vi "OE1022D Example All Data.vi"() -> ()   [LabVIEW 2022 SP3]
uses:
  <vilib>/Utility/file.llb/Write Delimited Spreadsheet (DBL).vi
panel:
  in  "OE1022D 2":refnum<visa-resource-name> caption="OE1022D"
  in  "Scanner Voltage":i32
  in  "File Path":path
  in  "Data Points":i32
  out "Waveform Chart":dbl[](graph)
  out "θh1 (°) 2":sgl caption="θh1 (deg)" format="%.2f"
  out "Rh1 2":sgl caption="Rh1 (Vrms)" format="%.3p"
  out "Yh1 2":sgl caption="Yh1 (Vrms)" format="%.3p"
  out "Xh1 2":sgl caption="Xh1 (Vrms)" format="%.3p"
  out "Xh2 2":sgl caption="Xh2 (Vrms)" format="%.3p"
  out "Yh2 2":sgl caption="Yh2 (Vrms)" format="%.3p"
  out "Rh2 2":sgl caption="Rh2 (Vrms)" format="%.3p"
  out "噪声 2":sgl caption="Noise(Vrms)" format="%.3p"
  out "频率 (Hz) 2":sgl caption="Freq (Hz)" format="%#.3f"
  out "θ (°) 2":sgl caption="θ (deg)" format="%.2f"
  out "R 2":sgl caption="R (Vrms)" format="%.3p"
  out "Y 2":sgl caption="Y (Vrms)" format="%.3p"
  out "θh2 (°) 2":sgl caption="θh2 (deg)" format="%.2f"
  out "X 2":sgl caption="X (Vrms)" format="%.3p"
  out "Yh1":sgl caption="Yh1 (Vrms)" format="%.3p"
  out "Xh1":sgl caption="Xh1 (Vrms)" format="%.3p"
  out "θh2 (°)":sgl caption="θh2 (deg)" format="%.2f"
  out "Yh2":sgl caption="Yh2 (Vrms)" format="%.3p"
  out "Xh2":sgl caption="Xh2 (Vrms)" format="%.3p"
  out "Rh2":sgl caption="Rh2 (Vrms)" format="%.3p"
  out "θh1 (°)":sgl caption="θh1 (deg)" format="%.2f"
  out "Rh1":sgl caption="Rh1 (Vrms)" format="%.3p"
  out "噪声":sgl caption="Noise(Vrms)" format="%.3p"
  out "频率 (Hz)":sgl caption="Freq (Hz)" format="%#.3f"
  out "θ (°)":sgl caption="θ (deg)" format="%.2f"
  out "Y":sgl caption="Y (Vrms)" format="%.3p"
  out "X":sgl caption="X (Vrms)" format="%.3p"
  out "R":sgl caption="R (Vrms)" format="%.3p"
  out "AUX-ADC2 (V)":sgl format="%.3f"
  out "AUX-ADC1 (V)":sgl format="%.3f"
  out "AUX-ADC3 (V)":sgl format="%.3f"
  out "AUX-ADC4 (V)":sgl format="%.3f"
  out "错误输出":errorcluster
  out "序列号":string
  # "input 0 for continous"
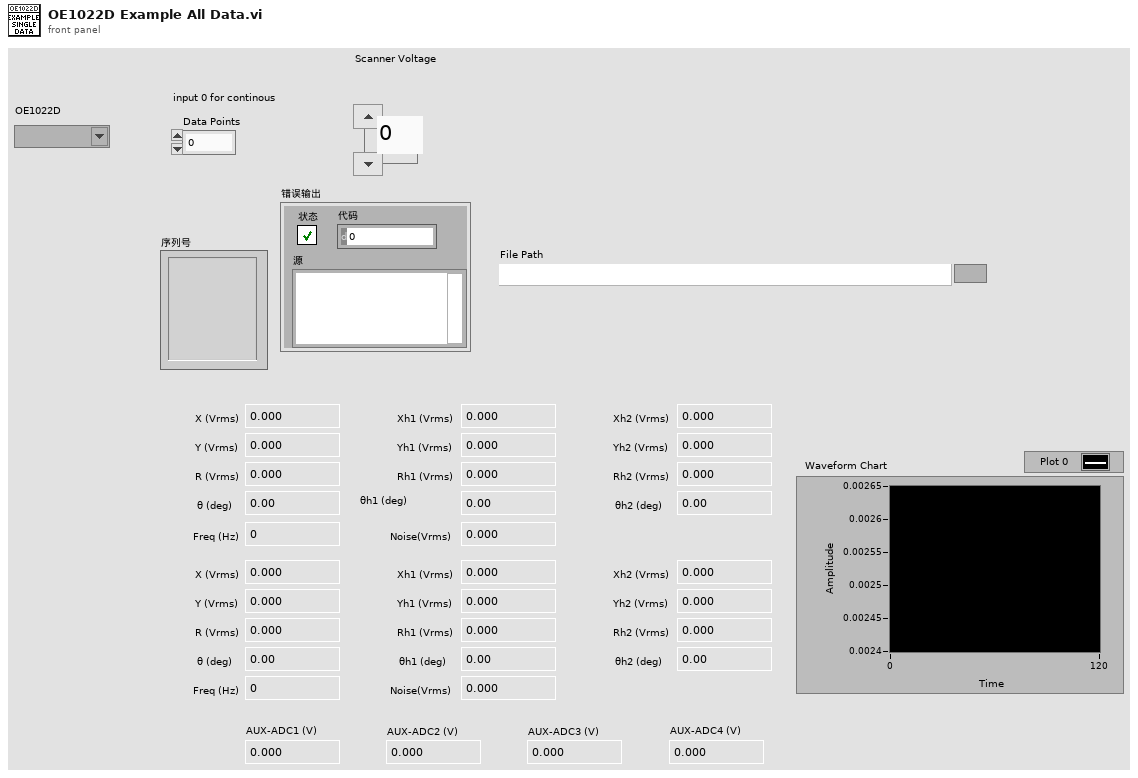
[diagram p1: front panel]
types:
  T1 = cluster{"AD1":dbl[], "AD2":dbl[], "AD3":dbl[], "AD4":dbl[]}
  T2 = cluster{"XB":dbl[], "YB":dbl[], "FrequencyB":dbl[], "NoiseB":dbl[], "Xh1B":dbl[], "Yh1B":dbl[], "Xh2B":dbl[], "Yh2B":dbl[], "Xh2B":dbl[]}
  T3 = cluster{"XA":dbl[], "YA":dbl[], "FrequencyA":dbl[], "NoiseA":dbl[], "Xh1A":dbl[], "Yh1A":dbl[], "Xh2A":dbl[], "Yh2A":dbl[]}
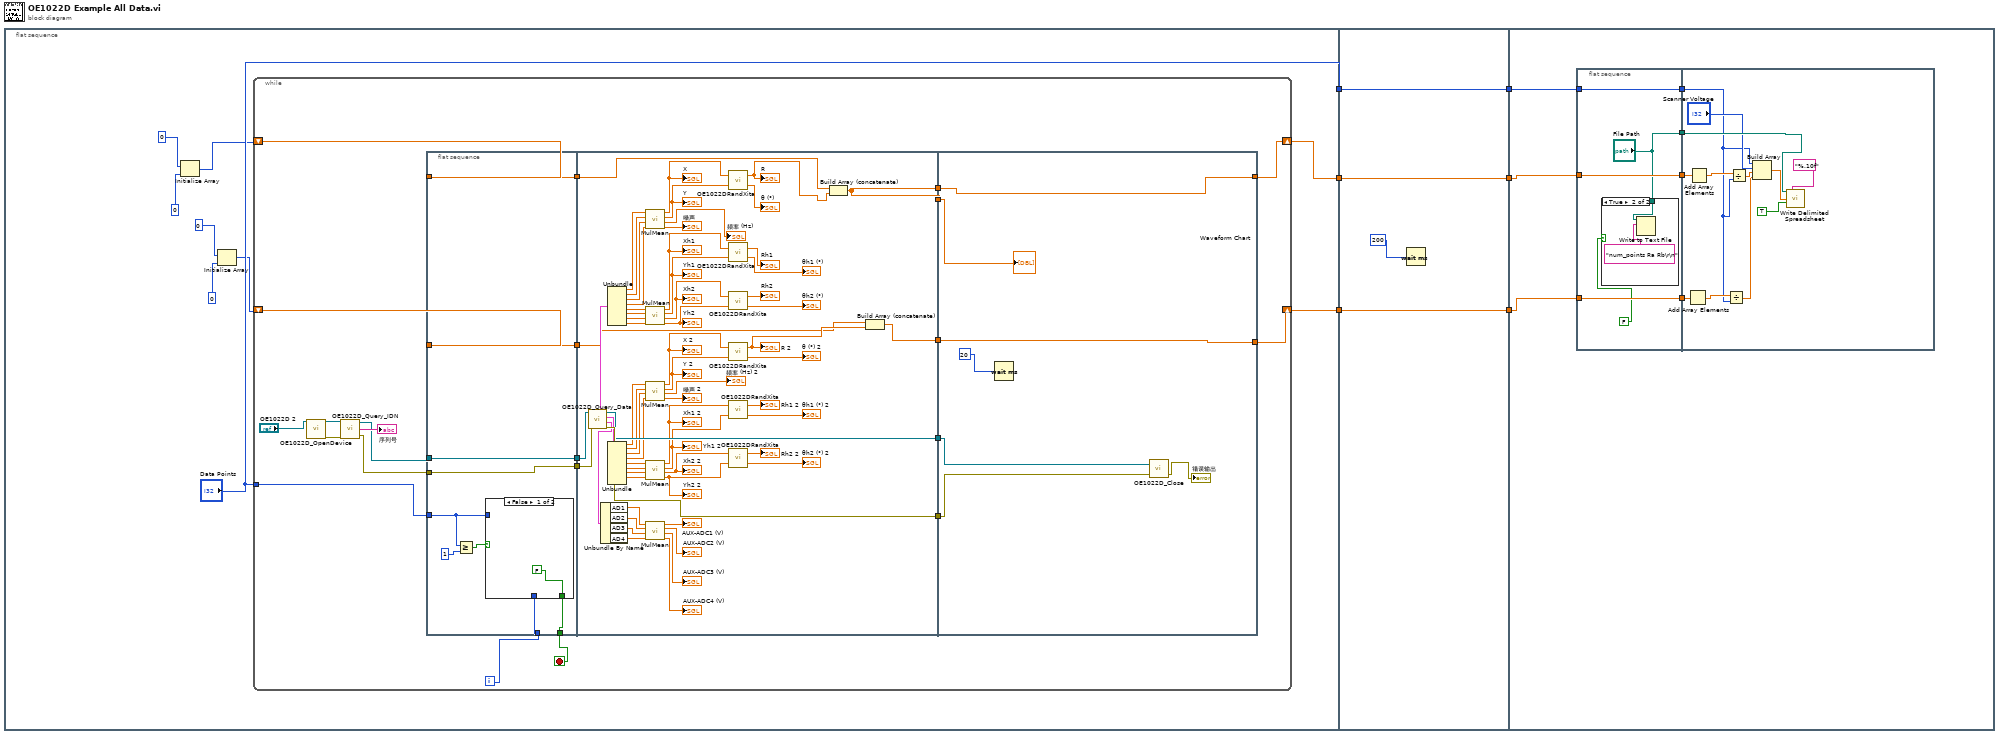
[diagram p0: block diagram]
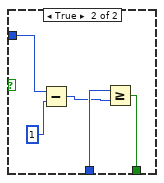
[diagram p2: hidden frame]
diagram:
  n1 = flat-sequence {
    tunnel: [w15] -> w6
    tunnel: [w14] -> w4
    tunnel: ["Data Points"] -> w2
    tunnel: w6 -> [w126]
    tunnel: [w126] -> w5
    tunnel: w4 -> [w125]
    tunnel: [w125] -> w3
    tunnel: w2 -> [w124]
    tunnel: [w124] -> w1
    tunnel: w5 -> [w129]
    tunnel: w3 -> [w128]
    tunnel: w1 -> [w127]
    frame #0 {
      n2 = Initialize Array(0, 0) -> (w12:i32[])
      n3 = Initialize Array(0, 0) -> (w7:i32[])
      n4 = while {
        shift-right: [w34] -> w15
        shift-left: w12 -> [w32]
        shift-right: [w30] -> w14
        shift-left: w7 -> [w29]
        tunnel: "Data Points" -> [w22]
        i -> [w24]
        stop <- w23 stop-if-true
        n5 = call "OE1022D_OpenDevice.vi"("VISA resource name"="OE1022D 2") -> ("VISA资源名称输出"=w20:refnum<visa-resource-name>, "错误输出"=w19:errorcluster)  [unwired: 17 in]
        n6 = call "OE1022D_Query_IDN.vi"("错误输入（无错误）"=w19, "VISA resource name"=w20) -> ("错误输出"=w17:errorcluster, "序列号"=→"序列号":string, "VISA resource name out"=w16:refnum<visa-resource-name>)  [unwired: 1 in]
        n7 = flat-sequence {
          tunnel: w29 -> [w44]
          tunnel: w32 -> [w45]
          tunnel: w16 -> [w46]
          tunnel: [w38] -> w28
          tunnel: [w46] -> w27
          tunnel: [w45] -> w26
          tunnel: [w44] -> w25
          tunnel: w24 -> [w43]
          tunnel: [w42] -> w23
          tunnel: w22 -> [w40]
          tunnel: w17 -> [w38]
          tunnel: [w113] -> w37
          tunnel: [w112] -> w36
          tunnel: [w56] -> w35
          tunnel: [w56] -> w33
          tunnel: [w53] -> w31
          tunnel: w28 -> [w115]
          tunnel: w27 -> [w114]
          tunnel: w26 -> [w57]
          tunnel: w25 -> [w54]
          tunnel: w37 -> [w118]
          tunnel: w36 -> [w117]
          tunnel: w35 -> [w121]
          tunnel: [w119] -> w34
          tunnel: w33 -> [w119]
          tunnel: w31 -> [w120]
          tunnel: [w120] -> w30
          frame #0 {
            n8 = Greater Or Equal?(x=w40, y=1) -> (x >= y?=w39:bool)
            n9 = case shown="False" w39 {
              tunnel: w43 -> [_ w52]
              tunnel: [FALSE w51] -> w42
              tunnel: w40 -> [_ w48]
              frame False {
              }
              frame True {
                n10 = Subtract(x=w48, y=1) -> (x-y=w49:i32)
                n11 = Greater Or Equal?(x=w52, y=w49) -> (x >= y?=w51:bool)
              }
            }
          }
          frame #1 {
            n12 = call "OE1022D_Query_Data.vi"("错误输入（无错误）"=w115, "VISA resource name"=w114) -> ("error out"=w113:errorcluster, "输出簇ADC"=w60:T1, "输出簇B"=w59:T2, "VISA resource name out"=w112:refnum<visa-resource-name>, "输出簇A"=w61:T3)  [unwired: 3 in]
            n13 = Unbundle By Name(w60) -> ("AD1"=w108:dbl[], "AD2"=w109:dbl[], "AD3"=w110:dbl[], "AD4"=w111:dbl[])
            n14 = Unbundle(w61) -> ("XA"=w66:dbl[], "YA"=w67:dbl[], "FrequencyA"=w68:dbl[], "NoiseA"=w69:dbl[], "Xh1A"=w75:dbl[], "Yh1A"=w76:dbl[], "Xh2A"=w77:dbl[], "Yh2A"=w78:dbl[])
            n15 = Unbundle(w59) -> ("XB"=w94:dbl[], "YB"=w93:dbl[], "FrequencyB"=w92:dbl[], "NoiseB"=w91:dbl[], "Xh1B"=w90:dbl[], "Yh1B"=w89:dbl[], "Xh2B"=w88:dbl[], "Yh2B"=w87:dbl[])  [unwired: 1 out]
            n16 = call "MulMean.vi"("IN 4"=w69, "IN 3"=w68, "IN 2"=w67, "IN 1"=w66) -> ("mean 4"=→"噪声":dbl, "mean 3"=→"频率 (Hz)":dbl, "mean 2"=w72:dbl, "mean 1"=w71:dbl)  [unwired: 4 in]
            "X" <- w71
            "Y" <- w72
            n17 = call "MulMean.vi"("IN 4"=w78, "IN 3"=w77, "IN 2"=w76, "IN 1"=w75) -> ("mean 4"=w84:dbl, "mean 3"=w83:dbl, "mean 2"=w80:dbl, "mean 1"=w79:dbl)  [unwired: 4 in]
            "Xh2" <- w83
            "Yh2" <- w84
            "Xh1" <- w79
            "Yh1" <- w80
            n18 = call "MulMean.vi"("IN 4"=w91, "IN 3"=w92, "IN 2"=w93, "IN 1"=w94) -> ("mean 4"=→"噪声 2":dbl, "mean 3"=→"频率 (Hz) 2":dbl, "mean 2"=w99:dbl, "mean 1"=w98:dbl)  [unwired: 4 in]
            "X 2" <- w98
            "Y 2" <- w99
            n19 = call "MulMean.vi"("IN 4"=w87, "IN 3"=w88, "IN 2"=w89, "IN 1"=w90) -> ("mean 4"=w105:dbl, "mean 3"=w104:dbl, "mean 2"=w101:dbl, "mean 1"=w100:dbl)  [unwired: 4 in]
            "Yh2 2" <- w105
            "Xh2 2" <- w104
            "Xh1 2" <- w100
            "Yh1 2" <- w101
            n20 = call "MulMean.vi"("IN 4"=w111, "IN 3"=w110, "IN 2"=w109, "IN 1"=w108) -> ("mean 4"=→"AUX-ADC4 (V)":dbl, "mean 3"=→"AUX-ADC3 (V)":dbl, "mean 2"=→"AUX-ADC2 (V)":dbl, "mean 1"=→"AUX-ADC1 (V)":dbl)  [unwired: 4 in]
            n21 = call "OE1022DRandXita.vi"("Y"=w72, "X"=w71) -> ("θ (°)"=→"θ (°)":dbl, "R"=w58:dbl)
            "R" <- w58
            n22 = call "OE1022DRandXita.vi"("Y"=w80, "X"=w79) -> ("θ (°)"=→"θh1 (°)":dbl, "R"=→"Rh1":dbl)
            n23 = call "OE1022DRandXita.vi"("Y"=w84, "X"=w83) -> ("θ (°)"=→"θh2 (°)":dbl, "R"=→"Rh2":dbl)
            n24 = call "OE1022DRandXita.vi"("Y"=w99, "X"=w98) -> ("θ (°)"=→"θ (°) 2":dbl, "R"=w55:dbl)
            "R 2" <- w55
            n25 = call "OE1022DRandXita.vi"("Y"=w101, "X"=w100) -> ("θ (°)"=→"θh1 (°) 2":dbl, "R"=→"Rh1 2":dbl)
            n26 = call "OE1022DRandXita.vi"("Y"=w105, "X"=w104) -> ("θ (°)"=→"θh2 (°) 2":dbl, "R"=→"Rh2 2":dbl)
            n27 = Build Array (concatenate)(w57, w58) -> (w56:dbl[])
            n28 = Build Array (concatenate)(w54, w55) -> (w53:dbl[])
          }
          frame #2 {
            n29 = Wait (ms)(milliseconds to wait=20) -> ()  [unwired: 1 out]
            n30 = call "OE1022D_Close.vi"("错误输入（无错误）"=w118, "VISA resource name"=w117) -> ("错误输出"=→"错误输出":errorcluster)  [unwired: 1 in]
            "Waveform Chart" <- w121
          }
        }
      }
    }
    frame #1 {
      n31 = Wait (ms)(milliseconds to wait=200) -> ()  [unwired: 1 out]
    }
    frame #2 {
      n32 = flat-sequence {
        tunnel: w127 -> [w136]
        tunnel: w128 -> [w137]
        tunnel: w129 -> [w138]
        tunnel: [w138] -> w133
        tunnel: [w137] -> w132
        tunnel: [w136] -> w131
        tunnel: ["File Path"] -> w130
        tunnel: w133 -> [w150]
        tunnel: w132 -> [w146]
        tunnel: w131 -> [w141]
        tunnel: w130 -> [w143]
        frame #0 {
          n33 = case shown="True" FALSE {
            tunnel: "File Path" -> [_ w140]
            frame False {
            }
            frame True {
              n34 = Write to Text File(file (use dialog)=w140, text="num_points Ra Rb\r\n") -> ()  [unwired: 2 in, 3 out]
            }
          }
        }
        frame #1 {
          n35 = Add Array Elements(numeric array=w146) -> (sum=w145:dbl)
          n36 = Add Array Elements(numeric array=w150) -> (sum=w149:dbl)
          n37 = Divide(x=w145, y=w141) -> (x/y=w144:dbl)
          n38 = Divide(x=w149, y=w141) -> (x/y=w148:dbl)
          n39 = Build Array(w141, "Scanner Voltage", w148, w144) -> (w147:dbl[])
          n40 = call-poly <vilib>:"Write Delimited Spreadsheet.vi"("file path (dialog if empty)"=w143, "format (%.3f)"="%.10f", "1D data"=w147, "append to file? (new file:F)"=TRUE) -> ()  [unwired: 10 in, 2 out]
        }
      }
    }
  }
